vi "多反-初定位.vi"(6 "显示搜索ROI":bool, 7 "反射镜数量":i32=9, 8 "镜像序列搜索半径":dbl=810.0, 9 "镜像序列搜索起始角":dbl=22.0, 10 "镜组中心位置":cluster{"X":i32, "Y":i32}={"X"=1200, "Y"=1050}, 11 "ImageIn":T4) -> (1 "产品搜索扇区":T1[](array[typedef]) {"End Angle" min=-90.0 max=90.0 step=1.0 format="%.2f"; "Start Angle" min=-90.0 max=90.0 step=1.0 format="%.2f"; "Center X" scale=0.0..1024.0}, 3 "ImageOut":T4)   [LabVIEW 2018]
uses:
  <vilib>/vision/Image Controls.llb/IMAQ Image.ctl
  <vilib>/vision/Measure.llb/Edge Options.ctl
  <vilib>/vision/Measure.llb/Edge Polarity.ctl
  <vilib>/vision/NI_Vision_Development_Module.lvlib
panel:
  in  "镜像产品底圆搜索特征半径":dbl=208.0
  in  "ROI中心产品搜索区域":T1={"Center X"=1260, "Center Y"=1010, "Inner Radius"=46, "Outer Radius"=143, "Start Angle"=0.0, "End Angle"=0.0} {"End Angle" min=-90.0 max=90.0 step=1.0 format="%.2f"; "Start Angle" min=-90.0 max=90.0 step=1.0 format="%.2f"; "Center X" scale=0.0..2500.0}
  in  "Edge Options":T2={"Edge Polarity"=2, "Kernel Size"=5, "Width"=9, "Minimum Edge Strength"=60.0, "Interpolation Type"=enum."Bilinear Fixed", "Data Processing Method"=enum."Average"} {"Edge Polarity" items=["All Edges", "Rising Edges", "Falling Edges"]; "Minimum Edge Strength" format="%.2f"; "Width" step=2; "Kernel Size" step=2}
  in  "单镜片区域搜索长度":i32=150
  in  "单镜片区域搜索宽度":i32=200
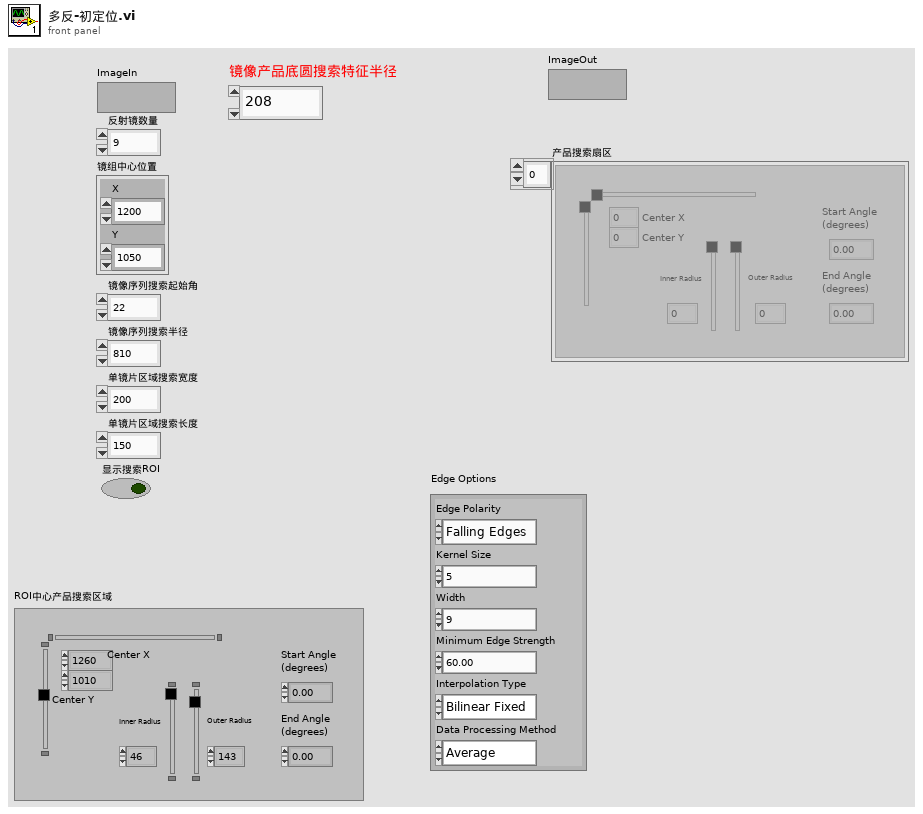
[diagram p1: front panel]
types:
  T1 = typedef "IMAQ Circle" = cluster{"Center X":i32, "Center Y":i32, "Inner Radius":i32, "Outer Radius":i32, "Start Angle":dbl, "End Angle":dbl}
  T2 = typedef "Edge Options.ctl" = cluster{"Edge Polarity":T3, "Kernel Size":u32, "Width":u32, "Minimum Edge Strength":sgl, "Interpolation Type":enum32{"Zero Order", "Bilinear", "Quadratic", "Cubic", "Bilinear Fixed"}, "Data Processing Method":enum32{"Average", "Median"}}
  T3 = typedef "Edge Polarity.ctl" = u32
  T4 = typedef "IMAQ Image.ctl" = refnum<image>
  T5 = enum16{"Get First Edge", "Get First + Last Edge", "Get All Edges", "Get Best Edge"}
  T6 = typedef "IMAQ Rectangle" = cluster{"Left":i32, "Top":i32, "Right":i32, "Bottom":i32, "Rotation":dbl}
  T7 = typedef "ROI Descriptor" = cluster{"Global Rectangle":i32[], "Contours":cluster{"ID":enum32{"External", "Internal"}, "Type":u32, "Coordinates":i32[]}[]}
  T8 = typedef "Edge New.ctl" = cluster{"Location (Pixel)":cluster{"X":sgl, "Y":sgl}, "Location (Real-World)":cluster{"X":sgl, "Y":sgl}, "Distance (Pixel)":dbl, "Distance (Real-World)":dbl, "Strength":dbl, "Noise":dbl, "Rising?":bool}
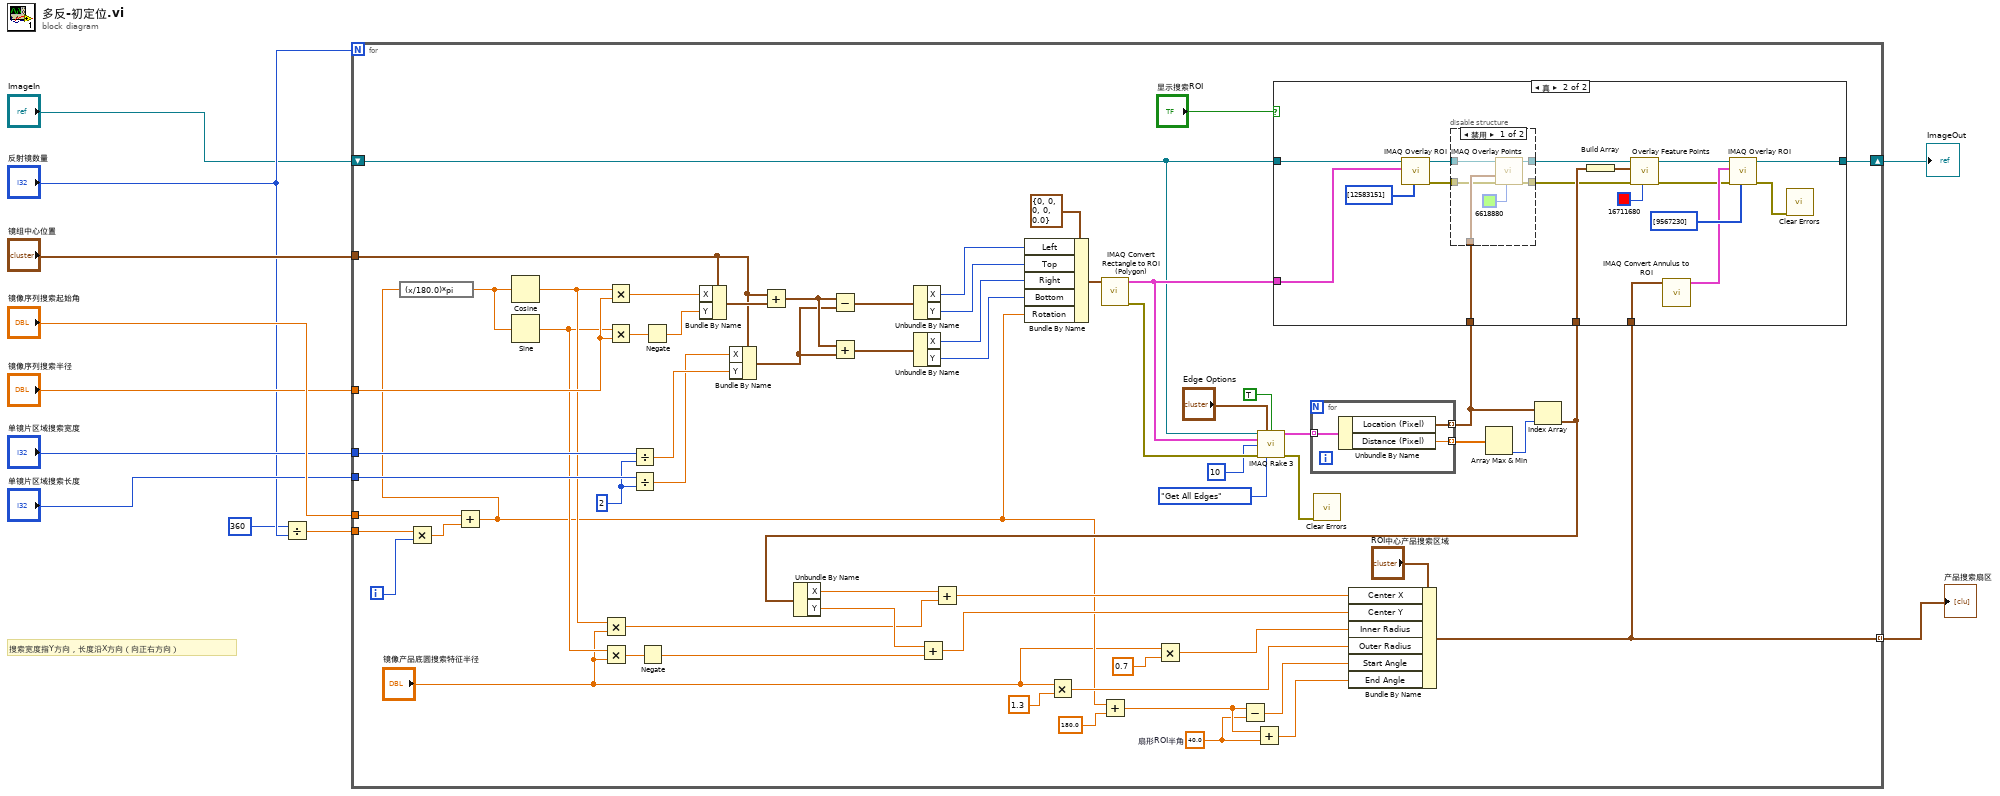
[diagram p0: block diagram]
diagram:
  # "搜索宽度指Y方向，长度沿X方向（向正右方向）"
  n1 = Divide(x=360, y="反射镜数量") -> (x/y=w4:dbl)
  n2 = for {
    N: "反射镜数量" -> [_]
    tunnel: "镜像序列搜索起始角" -> [w49]
    tunnel: "镜像序列搜索半径" -> [w73]
    tunnel: "单镜片区域搜索宽度" -> [w69]
    tunnel: "单镜片区域搜索长度" -> [w68]
    tunnel: "镜组中心位置" -> [w63]
    tunnel: w4 -> [w51]
    shift-right: [w37] -> w3
    shift-left: "ImageIn" -> [w47]
    tunnel: [w16] -> w1 mode=indexing
    i -> [w52]
    w12 = 40.0  # 扇形ROI半角
    w67 = 2 ("y")
    n3 = Multiply(x=w51, y=w52) -> (x*y=w50:dbl)
    n4 = Add(x=w49, y=w50) -> (x+y=w20:dbl)
    n5 = expression code="(x/180.0)*pi" ("degrees to radians")(w20) -> (w74:dbl)
    n6 = Cosine(x=w74) -> (cos(x)=w29:dbl)
    n7 = Sine(x=w74) -> (sin(x)=w28:dbl)
    n8 = Multiply(x=w29, y="镜像产品底圆搜索特征半径") -> (x*y=w24:dbl)
    n9 = Multiply(x=w28, y="镜像产品底圆搜索特征半径") -> (x*y=w30:dbl)
    n10 = Multiply(x=w29, y=w73) -> (x*y=w72:dbl)
    n11 = Multiply(x=w28, y=w73) -> (x*y=w62:dbl)
    n12 = Divide(x=w69, y=w67) -> (x/y=w66:dbl)
    n13 = Divide(x=w68, y=w67) -> (x/y=w65:dbl)
    n14 = Negate(x=w30) -> (-x=w23:dbl)
    n15 = Negate(x=w62) -> (-x=w61:dbl)
    n16 = Bundle By Name(cluster=w63, "X"=w72, "Y"=w61) -> (w71:cluster{"X":i32, "Y":i32})
    n17 = Bundle By Name(cluster=w63, "X"=w65, "Y"=w66) -> (w56:cluster{"X":i32, "Y":i32})
    n18 = Add(x=w63, y=w71) -> (x+y=w57:cluster{"X":i32, "Y":i32})
    n19 = Subtract(x=w57, y=w56) -> (x-y=w64:cluster{"X":i32, "Y":i32})
    n20 = Add(x=w57, y=w56) -> (x+y=w55:cluster{"X":i32, "Y":i32})
    n21 = Unbundle By Name(w64) -> ("X"=w60:i32, "Y"=w59:i32)
    n22 = Unbundle By Name(w55) -> ("X"=w54:i32, "Y"=w53:i32)
    n23 = Bundle By Name(cluster=T6 {"Left"=0, "Top"=0, "Right"=0, "Bottom"=0, "Rotation"=0.0} ("Rectangle"), "Left"=w60, "Top"=w59, "Right"=w54, "Bottom"=w53, "Rotation"=w20) -> (w58:T6)
    n24 = Multiply(x="镜像产品底圆搜索特征半径", y=1.3) -> (x*y=w31:dbl)
    n25 = call "IMAQ Convert Rectangle to ROI (Polygon)"("Rectangle"=w58) -> ("error out"=w44:errorcluster, "ROI Descriptor"=w48:T7)  [unwired: 7 in, 1 out]
    n26 = Add(x=w20, y=180.0) -> (x+y=w13:dbl)
    n27 = Multiply(x="镜像产品底圆搜索特征半径", y=0.7) -> (x*y=w17:dbl)
    n28 = Subtract(x=w13, y=w12) -> (x-y=w14:dbl)
    n29 = Add(x=w13, y=w12) -> (x+y=w35:dbl)
    n30 = call "IMAQ Rake 3"("Image"=w47, "Edge Options"="Edge Options", "Optimized Mode"=TRUE, "ROI Descriptor"=w48, "Step Size"=u32 10, "error in (no error)"=w44, "Process"=T5."Get All Edges") -> ("First Edges"=w41:T8[], "error out"=w15:errorcluster)  [unwired: 5 in, 2 out]
    n31 = for {
      tunnel: w41 -> [w104] mode=indexing
      tunnel: [w103] -> w39 mode=indexing
      tunnel: [w102] -> w40 mode=indexing
      n32 = Unbundle By Name(w104) -> ("Location (Pixel)"=w103:cluster{"X":sgl, "Y":sgl}, "Distance (Pixel)"=w102:dbl)
    }
    n33 = call <vilib>:"Clear Errors.vi"("error in (no error)"=w15) -> ()  [unwired: 5 in, 2 out]
    n34 = Array Max & Min(array=w40) -> (min index (indices)=w38:i32)  [unwired: 3 out]
    n35 = Index Array(array=w39, index=w38) -> (element=w27:cluster{"X":sgl, "Y":sgl})
    n36 = Unbundle By Name(w27) -> ("X"=w26:sgl, "Y"=w25:sgl)
    n37 = Add(x=w25, y=w23) -> (x+y=w21:dbl)
    n38 = Add(x=w26, y=w24) -> (x+y=w22:dbl)
    n39 = Bundle By Name(cluster="ROI中心产品搜索区域", "Center X"=w22, "Center Y"=w21, "Inner Radius"=w17, "Outer Radius"=w31, "Start Angle"=w14, "End Angle"=w35) -> (w16:T1)
    n40 = case shown="真" "显示搜索ROI" {
      tunnel: w48 -> [_ w93]
      tunnel: w47 -> [w75 w92]
      tunnel: w39 -> [_ w90]
      tunnel: [w75 w83] -> w37
      tunnel: w27 -> [_ w85]
      tunnel: w16 -> [_ w81]
      frame False {
      }
      frame True {
        n41 = call "IMAQ Overlay ROI"("Colors (Green)"=u32[] [12583151], "ROI Descriptor"=w93, "Image"=w92) -> ("error out"=w79:errorcluster, "Image Out"=w91:T4)  [unwired: 7 in]
        n42 = disable-structure shown="禁用" {
          disable-tunnel: w91 -> [w98 w101]
          disable-tunnel: w90 -> [w97 _]
          disable-tunnel: [w96 w101] -> w88
          disable-tunnel: w79 -> [w95 w100]
          disable-tunnel: [w94 w100] -> w78
          frame Disabled {
            n43 = call "IMAQ Overlay Points"("Color"=u32 6618880, "error in (no error)"=w95, "Array of Points"=w97, "Image"=w98) -> ("error out"=w94:errorcluster, "Image Out"=w96:T4)  [unwired: 6 in]
          }
          frame Enabled {
          }
        }
        n44 = Build Array(w85) -> (w86:cluster{"X":sgl, "Y":sgl}[])
        n45 = call "Overlay Feature Points.vi"("Color"=u32 16711680, "error in"=w78, "Feature Points"=w86, "Image"=w88) -> ("error out"=w77:errorcluster, "Image Out"=w84:T4)  [unwired: 6 in]
        n46 = call "IMAQ Convert Annulus to ROI"("Annulus"=w81) -> ("ROI Descriptor"=w80:T7)  [unwired: 8 in, 1 out]
        n47 = call "IMAQ Overlay ROI"("Colors (Green)"=u32[] [9567230], "error in (no error)"=w77, "ROI Descriptor"=w80, "Image"=w84) -> ("error out"=w76:errorcluster, "Image Out"=w83:T4)  [unwired: 6 in]
        n48 = call <vilib>:"Clear Errors.vi"("error in (no error)"=w76) -> ()  [unwired: 5 in, 2 out]
      }
    }
  }
  "ImageOut" <- w3
  "产品搜索扇区" <- w1
